vi "Analyze Data.vi"(8 "error in":errorcluster, 11 "nPAS in":refnum<class "nPAS.lvclass">) -> (0 "error out":errorcluster, 3 "nPAS out":refnum<class "nPAS.lvclass">)   [LabVIEW 2015, in "nPAS.lvclass"]
doc: "This is the core routine for PAS microphone data analysis. Here, the microphone data is retrieved from each of the cells. In both cases, the time domain signal will be transformed to the frequency domain. If the speaker is on (<B>Spk Pos</B> == TRUE), then the frequency domain signal will be squared to obtain the power and a Lorentzian will be fit to the data to retrieve the resonant characteristics of the cell. If the speaker is off (<B>Spk Pos</B> == FALSE), then the amplitude will be used to calculate the integrated area of the signal. In every case, the implementation has the ability to decimate the data for transmission of the waveforms over a network line."
uses:
  nPAS.lvclass
  nPAS.lvclass/nPAS.ctl
  Data/Nicholas Data.lvclass/Nicholas Data.ctl
  Accessors/Read Data DVR.vi
  Data/Write PAS.vi
  Reusable/PAS/Main/Get Speaker State.vi
  Reusable/PAS/Main/Read Data.vi
  Reusable/PAS/Data/Main/Write Current Cell.vi
  Reusable/PAS/Data/Main/Get f0.vi
  Reusable/PAS/Main/PAS.lvclass
  Reusable/PAS/Data/Main/PAS Data.lvclass
  Data/Nicholas Data.lvclass
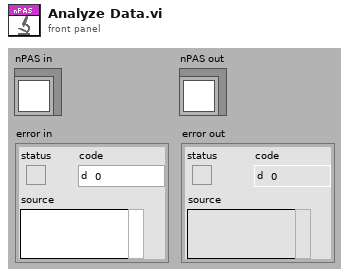
[diagram p1: front panel]
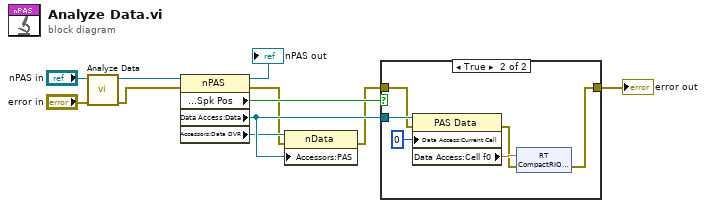
[diagram p0: block diagram]
diagram:
  n1 = call-parent "Analyze Data.vi"("error in"="error in", "PAS in"="nPAS in") -> ("error out"=w8:errorcluster, "PAS out"=w9:refnum<class "nPAS.lvclass">)  [unwired: 8 in]
  n2 = property class="nPAS"(reference=w9, error in=w8) -> (reference out=→"nPAS out":refnum<class "nPAS.lvclass">, error out=w2:errorcluster, "Data Access:Spk Pos"=w7:bool, "Data Access:Data"=w4:refnum<class "PAS Data.lvclass">, "Accessors:Data DVR"=w3:refnum<data-value>)
  n3 = property class="nData"(reference=w3, error in=w2, "Accessors:PAS"=w4) -> (error out=w1:errorcluster)  [unwired: 1 out]
  n4 = case shown="True" w7 {
    tunnel: w1 -> [w12 w13]
    tunnel: [w12 w15] -> w6
    tunnel: w4 -> [_ w14]
    frame False {
    }
    frame True {
      n5 = property class="PAS Data"(reference=w14, error in=w13, "Data Access:Current Cell"=0 ("Current Cell")) -> (error out=w16:errorcluster, "Data Access:Cell f0"=w17:sgl)  [unwired: 1 out]
      n6 = shared-variable "RT CompactRIO Target\\Nick SV.lvlib\\f0"(w17, error in=w16) -> (error out=w15:errorcluster)
    }
  }
  "error out" <- w6
